vi "Build-Window.vi"(8 "error in (no error)":errorcluster, 11 "WindowBuilder in":refnum<class "WindowBuilder.lvclass">) -> (0 "error out":errorcluster, 2 "Window":refnum<class "Window.lvclass">)   [LabVIEW 2024, in "GLF.lvlib" / "WindowBuilder.lvclass"]
uses:
  WindowBuilder.lvclass
  WindowBuilder.lvclass/WindowBuilder.ctl
  Window/Window.lvclass
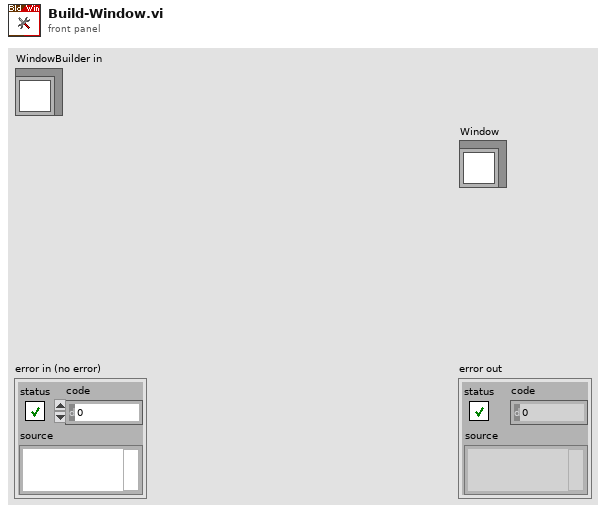
[diagram p1: front panel]
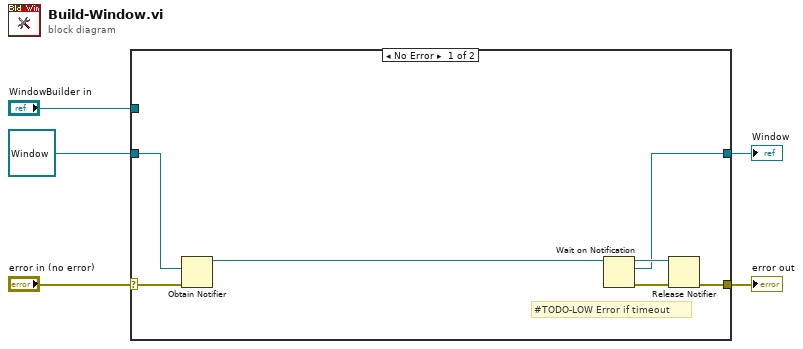
[diagram p0: block diagram]
diagram:
  n1 = case shown="No Error" "error in (no error)" {
    selector: "error in (no error)" -> [w12 w14]
    tunnel: [w6 w14] -> w4
    tunnel: "WindowBuilder in" -> [_ _]
    tunnel: [w7 w13] -> w2
    tunnel: refnum<class "Window.lvclass"> refnum ("Window") -> [w8 w13]
    frame No Error {
      # "#TODO-LOW Error if timeout"
      n2 = Obtain Notifier(notification data type=w8, error in (no error)=w12) -> (notifier out=w11:refnum<notifier>)  [unwired: 2 in, 2 out]
      n3 = Wait on Notification(notifier=w11) -> (notifier out=w10:refnum<notifier>, notification=w7:refnum<class "Window.lvclass">, error out=w9:errorcluster)  [unwired: 3 in, 1 out]
      n4 = Release Notifier(notifier=w10, error in (no error)=w9) -> (error out=w6:errorcluster)  [unwired: 1 in, 2 out]
    }
    frame Error {
    }
  }
  "error out" <- w4
  "Window" <- w2
